vi "Register.Get.vi"(8 "error in (no error)":errorcluster, 10 "Property":string="FPGA Register", 11 "Section Ref in":T1 format="%.0x") -> (0 "error out":errorcluster, 2 "Register":T2 {"Data Type" format="%.0x"}, 3 "Item Ref out":T1 format="%.0x")   [LabVIEW 2019, in "Fuel Injector Analysis Addon System Explorer.lvlib"]
uses:
  Fuel Injector Analysis Addon System Explorer.lvlib
  Shared/Types/Register.Info.ctl
  Shared/Types/FPGA Data Types.ctl
  <vilib>/NI VeriStand/Custom Device API/Custom Device Item Ref.ctl
  <vilib>/NI VeriStand/Custom Device API/Get Item Property (Variant).vi
  <vilib>/NI VeriStand/Custom Device API/Custom Device API.lvlib
  Shared/Fuel Injector Analysis Addon Shared.lvlib
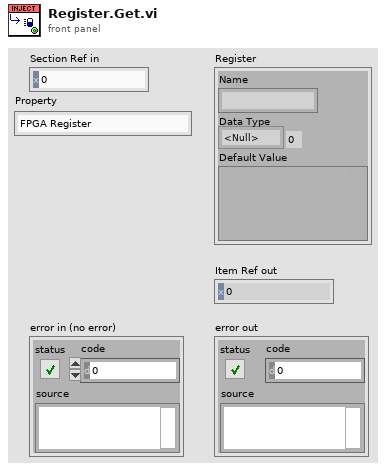
[diagram p1: front panel]
types:
  T1 = typedef "Custom Device API.lvlib/Custom Device Item Ref.ctl" = u64
  T2 = typedef "Fuel Injector Analysis Addon Shared.lvlib/Register.Info.ctl" = cluster{"Name":string, "Data Type":T3, "Default Value":variant}
  T3 = typedef "Fuel Injector Analysis Addon Shared.lvlib/FPGA Data Types.ctl" = enum8{"<Null>", "Injector.Core.Setting", "Injector.Global.Setting", "Injector.Mux.Setting", "Injector.Timing"}
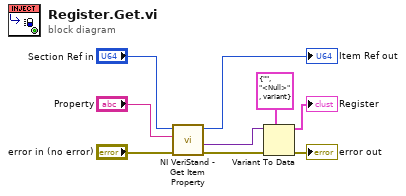
[diagram p0: block diagram]
diagram:
  n1 = call-poly <vilib>:"NI VeriStand - Get Item Property.vi"("error in (no error)"="error in (no error)", "Property Name"="Property", "Item Ref in"="Section Ref in") -> ("error out"=w6:errorcluster, "Value"=w5:variant, "Item Ref out"=→"Item Ref out":T1)  [unwired: 5 in, 1 out]
  n2 = Variant To Data(error in=w6, type=T2 {"Name"="", "Data Type"=enum."<Null>", "Default Value"=variant} ("Register"), Variant=w5) -> (data=→"Register":T2, error out=→"error out":errorcluster)
